vi "SeCrTS-DD signal names extracter.vi"(11 "input cluster":T1) -> (3 "Signal names":T2)   [LabVIEW 2022 SP3]
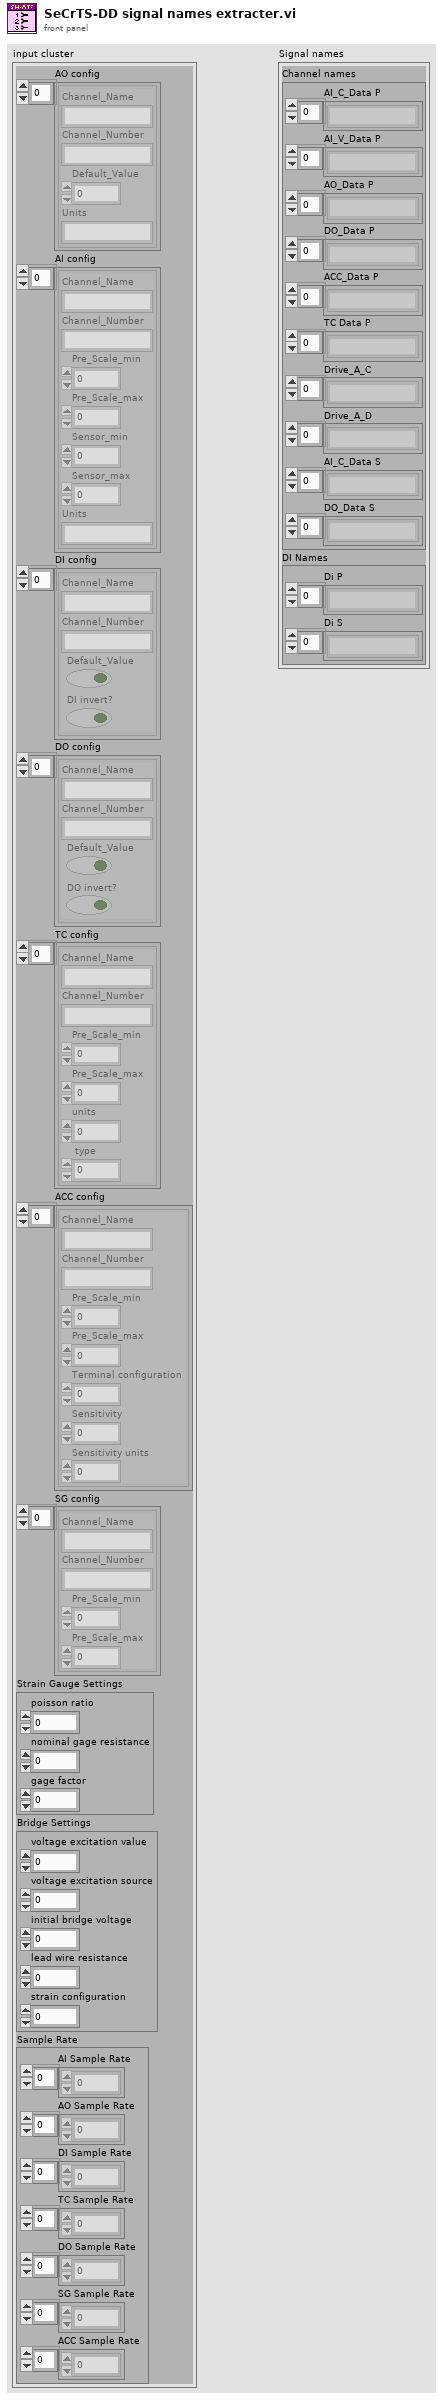
[diagram p1: front panel]
types:
  T1 = cluster{"AO config":cluster{"Channel_Name":string, "Channel_Number":string, "Default_Value":dbl, "Units":string}[], "AI config":cluster{"Channel_Name":string, "Channel_Number":string, "Pre_Scale_min":dbl, "Pre_Scale_max":dbl, "Sensor_min":dbl, "Sensor_max":dbl, "Units":string}[], "DI config":cluster{"Channel_Name":string, "Channel_Number":string, "Default_Value":bool, "DI invert?":bool}[], "DO config":cluster{"Channel_Name":string, "Channel_Number":string, "Default_Value":bool, "DO invert?":bool}[], "TC config":cluster{"Channel_Name":string, "Channel_Number":string, "Pre_Scale_min":dbl, "Pre_Scale_max":dbl, "units":i32, " type":i32}[], "ACC config":cluster{"Channel_Name":string, "Channel_Number":string, "Pre_Scale_min":dbl, "Pre_Scale_max":dbl, "Terminal configuration":i32, "Sensitivity":dbl, "Sensitivity units":i32}[], "SG config":cluster{"Channel_Name":string, "Channel_Number":string, "Pre_Scale_min":dbl, "Pre_Scale_max":dbl}[], "Strain Gauge Settings":cluster{"poisson ratio":dbl, "nominal gage resistance":dbl, "gage factor":dbl}, "Bridge Settings":cluster{"voltage excitation value":dbl, "voltage excitation source":i32, "initial bridge voltage":dbl, "lead wire resistance":dbl, "strain configuration":i32}, "Sample Rate":cluster{"AI Sample Rate":dbl[], "AO Sample Rate":dbl[], "DI Sample Rate":dbl[], "TC Sample Rate":dbl[], "DO Sample Rate":dbl[], "SG Sample Rate":dbl[], "ACC Sample Rate":dbl[]}}
  T2 = cluster{"Channel names":cluster{"AI_C_Data P":string[], "AI_V_Data P":string[], "AO_Data P":string[], "DO_Data P":string[], "ACC_Data P":string[], "TC Data P":string[], "Drive_A_C":string[], "Drive_A_D":string[], "AI_C_Data S":string[], "DO_Data S":string[]}, "DI Names":cluster{"Di P":string[], "Di S":string[]}}
  T3 = cluster{"Channel_Name":string, "Channel_Number":string, "Default_Value":dbl, "Units":string}[]
  T4 = cluster{"Channel_Name":string, "Channel_Number":string, "Pre_Scale_min":dbl, "Pre_Scale_max":dbl, "Sensor_min":dbl, "Sensor_max":dbl, "Units":string}[]
  T5 = cluster{"Channel_Name":string, "Channel_Number":string, "Default_Value":bool, "DI invert?":bool}[]
  T6 = cluster{"Channel_Name":string, "Channel_Number":string, "Default_Value":bool, "DO invert?":bool}[]
  T7 = cluster{"Channel_Name":string, "Channel_Number":string, "Pre_Scale_min":dbl, "Pre_Scale_max":dbl, "units":i32, " type":i32}[]
  T8 = cluster{"Channel_Name":string, "Channel_Number":string, "Pre_Scale_min":dbl, "Pre_Scale_max":dbl, "Terminal configuration":i32, "Sensitivity":dbl, "Sensitivity units":i32}[]
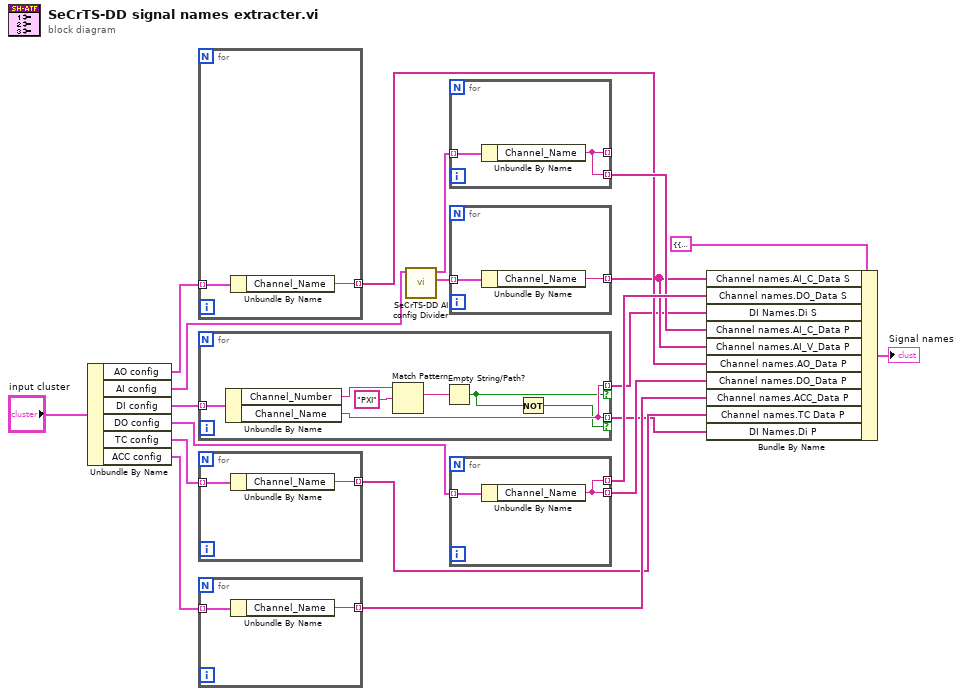
[diagram p0: block diagram]
diagram:
  n1 = Unbundle By Name("input cluster") -> ("AO config"=w13:T3, "AI config"=w18:T4, "DI config"=w14:T5, "DO config"=w15:T6, "TC config"=w16:T7, "ACC config"=w17:T8)
  n2 = for {
    tunnel: w13 -> [w22] mode=indexing
    tunnel: [w21] -> w9 mode=indexing
    n3 = Unbundle By Name(w22) -> ("Channel_Name"=w21:string)
  }
  n4 = for {
    tunnel: w14 -> [w29] mode=indexing
    tunnel: [w25] -> w1 mode=indexing if=w24
    tunnel: [w25] -> w2 mode=indexing if=w23
    n5 = Unbundle By Name(w29) -> ("Channel_Number"=w28:string, "Channel_Name"=w25:string)
    n6 = Match Pattern(string=w28, regular expression="PXI") -> (match substring=w26:string)  [unwired: 1 in, 3 out]
    n7 = Empty String/Path?(string/path=w26) -> (empty?=w24:bool)
    n8 = Not(x=w24) -> (.not. x?=w23:bool)
  }
  n9 = for {
    tunnel: [w31] -> w6 mode=indexing
    tunnel: w16 -> [w30] mode=indexing
    n10 = Unbundle By Name(w30) -> ("Channel_Name"=w31:string)
  }
  n11 = for {
    tunnel: w17 -> [w33] mode=indexing
    tunnel: [w32] -> w7 mode=indexing
    n12 = Unbundle By Name(w33) -> ("Channel_Name"=w32:string)
  }
  n13 = call "SeCrTS-DD AI config Divider.vi"("AI config"=w18) -> ("AI V"=w20:T4, "AI C"=w19:T4)  [unwired: 9 in]
  n14 = for {
    tunnel: w19 -> [w35] mode=indexing
    tunnel: [w34] -> w10 mode=indexing
    tunnel: [w34] -> _ mode=indexing
    n15 = Unbundle By Name(w35) -> ("Channel_Name"=w34:string)
  }
  n16 = for {
    tunnel: w20 -> [w37] mode=indexing
    tunnel: [w36] -> w4 mode=indexing
    n17 = Unbundle By Name(w37) -> ("Channel_Name"=w36:string)
  }
  n18 = for {
    tunnel: w15 -> [w39] mode=indexing
    tunnel: [w38] -> w8 mode=indexing
    tunnel: [w38] -> w11 mode=indexing
    n19 = Unbundle By Name(w39) -> ("Channel_Name"=w38:string)
  }
  n20 = Bundle By Name(cluster=T2 {"Channel names"={"AI_C_Data P"=[], "AI_V_Data P"=[], "AO_Data P"=[], "DO_Data P"=[], "ACC_Data P"=[], "TC Data P"=[], "Drive_A_C"=[], "Drive_A_D"=[], "AI_C_Data S"=[], "DO_Data S"=[]}, "DI Names"={"Di P"=[], "Di S"=[]}} ("Signal names"), "Channel names.AI_C_Data S"=w4, "Channel names.DO_Data S"=w11, "DI Names.Di S"=w1, "Channel names.AI_C_Data P"=w10, "Channel names.AI_V_Data P"=w4, "Channel names.AO_Data P"=w9, "Channel names.DO_Data P"=w8, "Channel names.ACC_Data P"=w7, "Channel names.TC Data P"=w6, "DI Names.Di P"=w2) -> (→"Signal names":T2)
